vi "Configure Trigger.vi"   [LabVIEW 2021, in "Siglent SDS 1000 2000 Series.lvlib"]
doc: "Selects the type of trigger: Edge trigger, Glitch trigger, TV trigger and Slope trigger."
uses:
  <instrlib>/Siglent SDS 1000 2000 Series/Siglent SDS 1000 2000 Series.lvlib
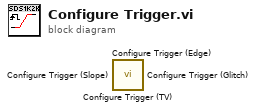
[diagram p0: block diagram]
diagram:
  n1 = call <instrlib>:"Configure Trigger (TV).vi"() -> ()  [unwired: 14 in, 2 out]
  n2 = call <instrlib>:"Configure Trigger (Edge).vi"() -> ()  [unwired: 14 in, 2 out]
  n3 = call <instrlib>:"Configure Trigger (Slope).vi"() -> ()  [unwired: 14 in, 2 out]
  n4 = call <instrlib>:"Configure Trigger (Glitch).vi"() -> ()  [unwired: 14 in, 2 out]
